vi "PSVCH_Constant String Check.vi"(7 "String":string) -> (6 "Constant?":bool, 8 "Type":string, 10 "Value":variant)   [LabVIEW 2016]
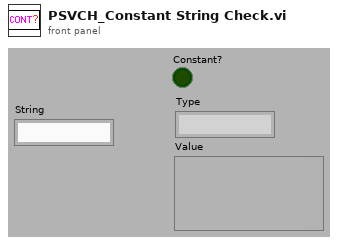
[diagram p1: front panel]
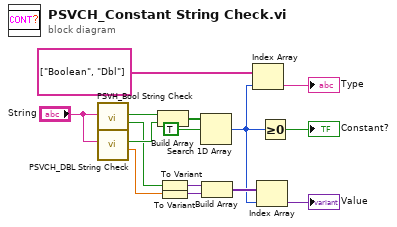
[diagram p0: block diagram]
diagram:
  n1 = call "PSVH_Bool String Check.vi"("Bool Str"="String") -> ("Boolean"=w7:bool, "Bool?"=w13:bool)  [unwired: 9 in]
  n2 = call "PSVCH_DBL String Check.vi"("Num Str"="String") -> ("Number"=w6:dbl, "Num?"=w14:bool)  [unwired: 9 in]
  n3 = Build Array(w13, w14) -> (w12:bool[])
  n4 = To Variant(anything=w7) -> (Variant=w5:variant)
  n5 = To Variant(anything=w6) -> (Variant=w4:variant)
  n6 = Search 1D Array(1D array=w12, element=TRUE) -> (index of element=w2:i32)  [unwired: 1 in]
  n7 = Build Array(w5, w4) -> (w3:variant[])
  n8 = Index Array(array=string[] ["Boolean", "Dbl"], index=w2) -> (element=→"Type":string)
  n9 = Index Array(array=w3, index=w2) -> (element=→"Value":variant)
  n10 = Greater Or Equal To 0?(x=w2) -> (x >= 0?=→"Constant?":bool)
